vi "Raycaster_CalcCameraX.vi"() -> (3 "CameraX":fxp<+/-,32,16>[](array[numeric])=[-1.0, -0.9950103759765625, -0.9900054931640625, -0.9850006103515625, -0.980010986328125, -0.975006103515625, -0.970001220703125, -0.9650115966796875, -0.9600067138671875, -0.9550018310546875, -0.95001220703125, -0.94500732421875, -0.94000244140625, -0.9350128173828125, -0.9300079345703125, -0.9250030517578125, -0.920013427734375, -0.915008544921875, -0.910003662109375, -0.9050140380859375, -0.9000091552734375, -0.8950042724609375, -0.8900146484375, -0.885009765625, -0.8800048828125, -0.875, -0.8700103759765625, -0.8650054931640625, -0.8600006103515625, -0.855010986328125, -0.850006103515625, -0.845001220703125, -0.8400115966796875, -0.8350067138671875, -0.8300018310546875, -0.82501220703125, -0.82000732421875, -0.81500244140625, -0.8100128173828125, -0.8050079345703125, -0.8000030517578125, -0.795013427734375, -0.790008544921875, -0.785003662109375, -0.7800140380859375, -0.7750091552734375, -0.7700042724609375, -0.7650146484375, -0.760009765625, -0.7550048828125, -0.75, -0.7450103759765625, -0.7400054931640625, -0.7350006103515625, -0.730010986328125, -0.725006103515625, -0.720001220703125, -0.7150115966796875, -0.7100067138671875, -0.7050018310546875, -0.70001220703125, -0.69500732421875, -0.69000244140625, -0.6850128173828125, -0.6800079345703125, -0.6750030517578125, -0.670013427734375, -0.665008544921875, -0.660003662109375, -0.6550140380859375, -0.6500091552734375, -0.6450042724609375, -0.6400146484375, -0.635009765625, -0.6300048828125, -0.625, -0.6200103759765625, -0.6150054931640625, -0.6100006103515625, -0.605010986328125, -0.600006103515625, -0.595001220703125, -0.5900115966796875, -0.5850067138671875, -0.5800018310546875, -0.57501220703125, -0.57000732421875, -0.56500244140625, -0.5600128173828125, -0.5550079345703125, -0.5500030517578125, -0.545013427734375, -0.540008544921875, -0.535003662109375, -0.5300140380859375, -0.5250091552734375, -0.5200042724609375, -0.5150146484375, -0.510009765625, -0.5050048828125, -0.5, -0.4950103759765625, -0.4900054931640625, -0.4850006103515625, -0.480010986328125, -0.475006103515625, -0.470001220703125, -0.4650115966796875, -0.4600067138671875, -0.4550018310546875, -0.45001220703125, -0.44500732421875, -0.44000244140625, -0.4350128173828125, -0.4300079345703125, -0.4250030517578125, -0.420013427734375, -0.415008544921875, -0.410003662109375, -0.4050140380859375, -0.4000091552734375, -0.3950042724609375, -0.3900146484375, -0.385009765625, -0.3800048828125, -0.375, -0.3700103759765625, -0.3650054931640625, -0.3600006103515625, -0.355010986328125, -0.350006103515625, -0.345001220703125, -0.3400115966796875, -0.3350067138671875, -0.3300018310546875, -0.32501220703125, -0.32000732421875, -0.31500244140625, -0.3100128173828125, -0.3050079345703125, -0.3000030517578125, -0.295013427734375, -0.290008544921875, -0.285003662109375, -0.2800140380859375, -0.2750091552734375, -0.2700042724609375, -0.2650146484375, -0.260009765625, -0.2550048828125, -0.25, -0.2450103759765625, -0.2400054931640625, -0.2350006103515625, -0.230010986328125, -0.225006103515625, -0.220001220703125, -0.2150115966796875, -0.2100067138671875, -0.2050018310546875, -0.20001220703125, -0.19500732421875, -0.19000244140625, -0.1850128173828125, -0.1800079345703125, -0.1750030517578125, -0.170013427734375, -0.165008544921875, -0.160003662109375, -0.1550140380859375, -0.1500091552734375, -0.1450042724609375, -0.1400146484375, -0.135009765625, -0.1300048828125, -0.125, -0.1200103759765625, -0.1150054931640625, -0.1100006103515625, -0.105010986328125, -0.100006103515625, -0.095001220703125, -0.0900115966796875, -0.0850067138671875, -0.0800018310546875, -0.07501220703125, -0.07000732421875, -0.06500244140625, -0.0600128173828125, -0.0550079345703125, -0.0500030517578125, -0.045013427734375, -0.040008544921875, -0.035003662109375, -0.0300140380859375, -0.0250091552734375, -0.0200042724609375, -0.0150146484375, -0.010009765625, -0.0050048828125, 0.0, 0.0049896240234375, 0.0099945068359375, 0.0149993896484375, 0.019989013671875, 0.024993896484375, 0.029998779296875, 0.0349884033203125, 0.0399932861328125, 0.0449981689453125, 0.04998779296875, 0.05499267578125, 0.05999755859375, 0.0649871826171875, 0.0699920654296875, 0.0749969482421875, 0.079986572265625, 0.084991455078125, 0.089996337890625, 0.0949859619140625, 0.0999908447265625, 0.1049957275390625, 0.1099853515625, 0.114990234375, 0.1199951171875, 0.125, 0.1299896240234375, 0.1349945068359375, 0.1399993896484375, 0.144989013671875, 0.149993896484375, 0.154998779296875, 0.1599884033203125, 0.1649932861328125, 0.1699981689453125, 0.17498779296875, 0.17999267578125, 0.18499755859375, 0.1899871826171875, 0.1949920654296875, 0.1999969482421875, 0.204986572265625, 0.209991455078125, 0.214996337890625, 0.2199859619140625, 0.2249908447265625, 0.2299957275390625, 0.2349853515625, 0.239990234375, 0.2449951171875, 0.25, 0.2549896240234375, 0.2599945068359375, 0.2649993896484375, 0.269989013671875, 0.274993896484375, 0.279998779296875, 0.2849884033203125, 0.2899932861328125, 0.2949981689453125, 0.29998779296875, 0.30499267578125, 0.30999755859375, 0.3149871826171875, 0.3199920654296875, 0.3249969482421875, 0.329986572265625, 0.334991455078125, 0.339996337890625, 0.3449859619140625, 0.3499908447265625, 0.3549957275390625, 0.3599853515625, 0.364990234375, 0.3699951171875, 0.375, 0.3799896240234375, 0.3849945068359375, 0.3899993896484375, 0.394989013671875, 0.399993896484375, 0.404998779296875, 0.4099884033203125, 0.4149932861328125, 0.4199981689453125, 0.42498779296875, 0.42999267578125, 0.43499755859375, 0.4399871826171875, 0.4449920654296875, 0.4499969482421875, 0.454986572265625, 0.459991455078125, 0.464996337890625, 0.4699859619140625, 0.4749908447265625, 0.4799957275390625, 0.4849853515625, 0.489990234375, 0.4949951171875, 0.5, 0.5049896240234375, 0.5099945068359375, 0.5149993896484375, 0.519989013671875, 0.524993896484375, 0.529998779296875, 0.5349884033203125, 0.5399932861328125, 0.5449981689453125, 0.54998779296875, 0.55499267578125, 0.55999755859375, 0.5649871826171875, 0.5699920654296875, 0.5749969482421875, 0.579986572265625, 0.584991455078125, 0.589996337890625, 0.5949859619140625, 0.5999908447265625, 0.6049957275390625, 0.6099853515625, 0.614990234375, 0.6199951171875, 0.625, 0.6299896240234375, 0.6349945068359375, 0.6399993896484375, 0.644989013671875, 0.649993896484375, 0.654998779296875, 0.6599884033203125, 0.6649932861328125, 0.6699981689453125, 0.67498779296875, 0.67999267578125, 0.68499755859375, 0.6899871826171875, 0.6949920654296875, 0.6999969482421875, 0.704986572265625, 0.709991455078125, 0.714996337890625, 0.7199859619140625, 0.7249908447265625, 0.7299957275390625, 0.7349853515625, 0.739990234375, 0.7449951171875, 0.75, 0.7549896240234375, 0.7599945068359375, 0.7649993896484375, 0.769989013671875, 0.774993896484375, 0.779998779296875, 0.7849884033203125, 0.7899932861328125, 0.7949981689453125, 0.79998779296875, 0.80499267578125, 0.80999755859375, 0.8149871826171875, 0.8199920654296875, 0.8249969482421875, 0.829986572265625, 0.834991455078125, 0.839996337890625, 0.8449859619140625, 0.8499908447265625, 0.8549957275390625, 0.8599853515625, 0.864990234375, 0.8699951171875, 0.875, 0.8799896240234375, 0.8849945068359375, 0.8899993896484375, 0.894989013671875, 0.899993896484375, 0.904998779296875, 0.9099884033203125, 0.9149932861328125, 0.9199981689453125, 0.92498779296875, 0.92999267578125, 0.93499755859375, 0.9399871826171875, 0.9449920654296875, 0.9499969482421875, 0.954986572265625, 0.959991455078125, 0.964996337890625, 0.9699859619140625, 0.9749908447265625, 0.9799957275390625, 0.9849853515625, 0.989990234375, 0.9949951171875])   [LabVIEW 2020]
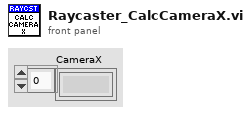
[diagram p1: front panel]
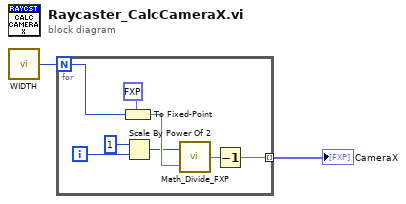
[diagram p0: block diagram]
diagram:
  n1 = call "WIDTH.vi"() -> ("WIDTH"=w1:i16)
  n2 = for {
    N: w1 -> [w3]
    tunnel: [w7] -> w2 mode=indexing
    i -> [w6]
    n3 = To Fixed-Point(fixed-point type=fxp<+/-,32,16> 0.0, number=w3) -> (fixed-point=w9:fxp<+/-,32,16>)
    n4 = Scale By Power Of 2(n=i16 1, x=w6) -> (x*2^n=w4:i32)
    n5 = call "Math_Divide_FXP.vi"("y"=w9, "x"=w4) -> ("x*y"=w10:fxp<+/-,32,16>)
    n6 = Decrement(x=w10) -> (x-1=w7:fxp<+/-,32,16>)
  }
  "CameraX" <- w2
